vi "Make empty strings null.vi"(11 "JSON Input":string) -> (3 "<JSON>":string)   [LabVIEW 2024, in "JSONtext.lvlib"]
doc: "Make empty input (or all whitespace)count as null"
uses:
  JSONtext.lvlib
  JDP Utility.lvlib
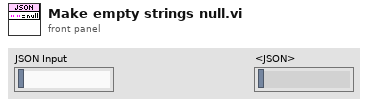
[diagram p1: front panel]
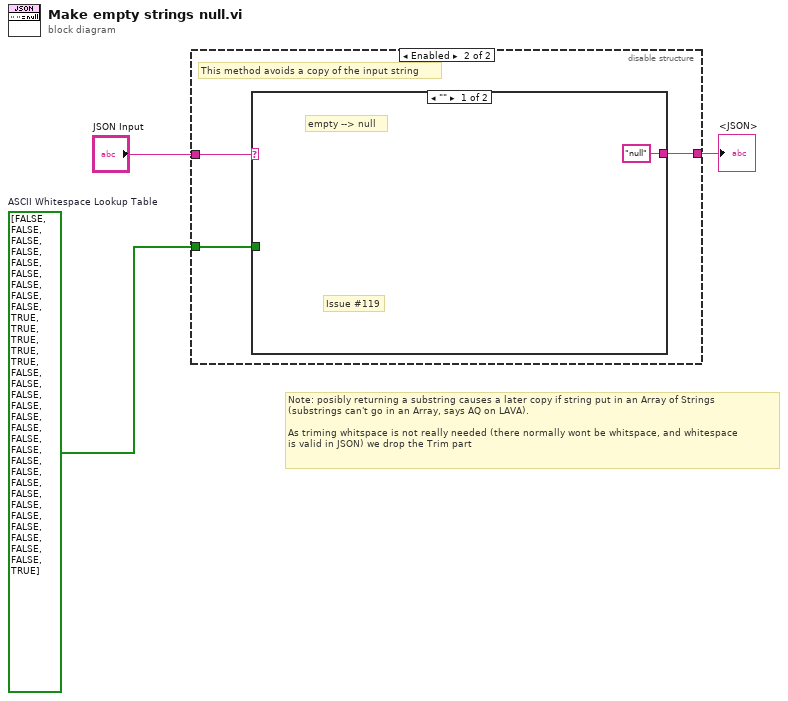
[diagram p0: block diagram]
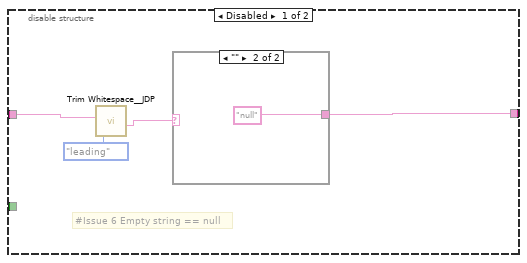
[diagram p2: hidden frame]
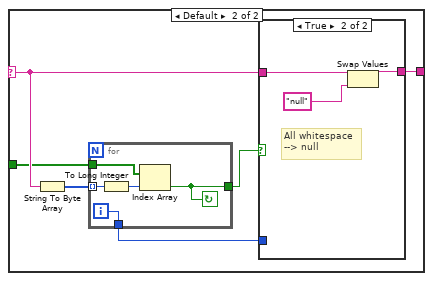
[diagram p4: hidden frame]
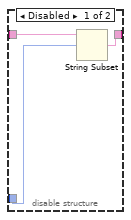
[diagram p6: hidden frame]
diagram:
  w1 = bool[] [FALSE, FALSE, FALSE, FALSE, FALSE, FALSE, FALSE, FALSE, FALSE, TRUE, TRUE, TRUE, TRUE, TRUE, FALSE, FALSE, FALSE, FALSE, FALSE, FALSE, FALSE, FALSE, FALSE, FALSE, FALSE, FALSE, FALSE, FALSE, FALSE, FALSE, FALSE, FALSE, TRUE]  # ASCII Whitespace Lookup Table
  # "Note: posibly returning a substring causes a later copy if string put in an Array of Strings\n(substrings can't go in an Array, says AQ on LAVA).\n\nAs triming whitspace is not really needed (there normally wont be whitspace, and whitespace\nis valid in JSON) we drop the Trim part"
  n1 = disable-structure shown="Enabled" {
    disable-tunnel: "JSON Input" -> [w7 w12]
    disable-tunnel: [w5 w11] -> w2
    disable-tunnel: w1 -> [_ w10]
    frame Disabled {
      # "#Issue 6 Empty string == null"
      n2 = call "Trim Whitespace__JDP.vi"("Remove (leading and trailing)"=enum16{"leading", "trailing", "both"}."leading", "String in"=w7) -> ("String out"=w6:string)  [unwired: 5 in]
      n3 = case shown="\"\"" w6 {
        selector: w6 -> [w8 _]
        tunnel: [w8 "null"] -> w5
        frame Default {
        }
        frame "" {
        }
      }
    }
    frame Enabled {
      # "This method avoids a copy of the input string"
      n4 = case shown="\"\"" w12 {
        selector: w12 -> [_ w18]
        tunnel: ["null" w17] -> w11
        tunnel: w10 -> [_ w14]
        frame "" {
          # "Issue #119"
          # "empty --> null"
        }
        frame Default {
          n5 = String To Byte Array(string=w18) -> (unsigned byte array=w19:u8[])
          n6 = for {
            tunnel: w19 -> [w34] mode=indexing
            tunnel: [w32] -> w16
            tunnel: [w31] -> w15
            tunnel: w14 -> [w30]
            i -> [w31]
            stop <- w32 continue-if-true
            n7 = To Long Integer(number=w34) -> (32bit integer=w33:i32)
            n8 = Index Array(array=w30, index=w33) -> (element=w32:bool)
          }
          n9 = case shown="True" w16 {
            tunnel: w18 -> [w21 w29]
            tunnel: [w22 w28] -> w17
            tunnel: w15 -> [w20 _]
            frame False {
              n10 = disable-structure shown="Enabled" {
                disable-tunnel: [w25 w26] -> w22
                disable-tunnel: w21 -> [w24 w26]
                disable-tunnel: w20 -> [w23 _]
                frame Disabled {
                  n11 = String Subset(string=w24, offset (0)=w23) -> (substring=w25:string)  [unwired: 1 in]
                }
                frame Enabled {
                }
              }
            }
            frame True {
              # "All whitespace\n--> null"
              n12 = Swap Values(12:w29, 14:"null") -> (1:w28:string)  [unwired: 1 in, 1 out]
            }
          }
        }
      }
    }
  }
  "<JSON>" <- w2
